vi "CRC.vi"(9 "Len":u8, 11 "u8Buf":u8[](array[numeric]) format="%x") -> (3 "CRC":u16 format="%x")   [LabVIEW 2018]
panel:
  # "CRC-16 Calculation"
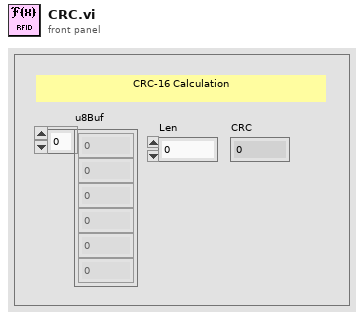
[diagram p1: front panel]
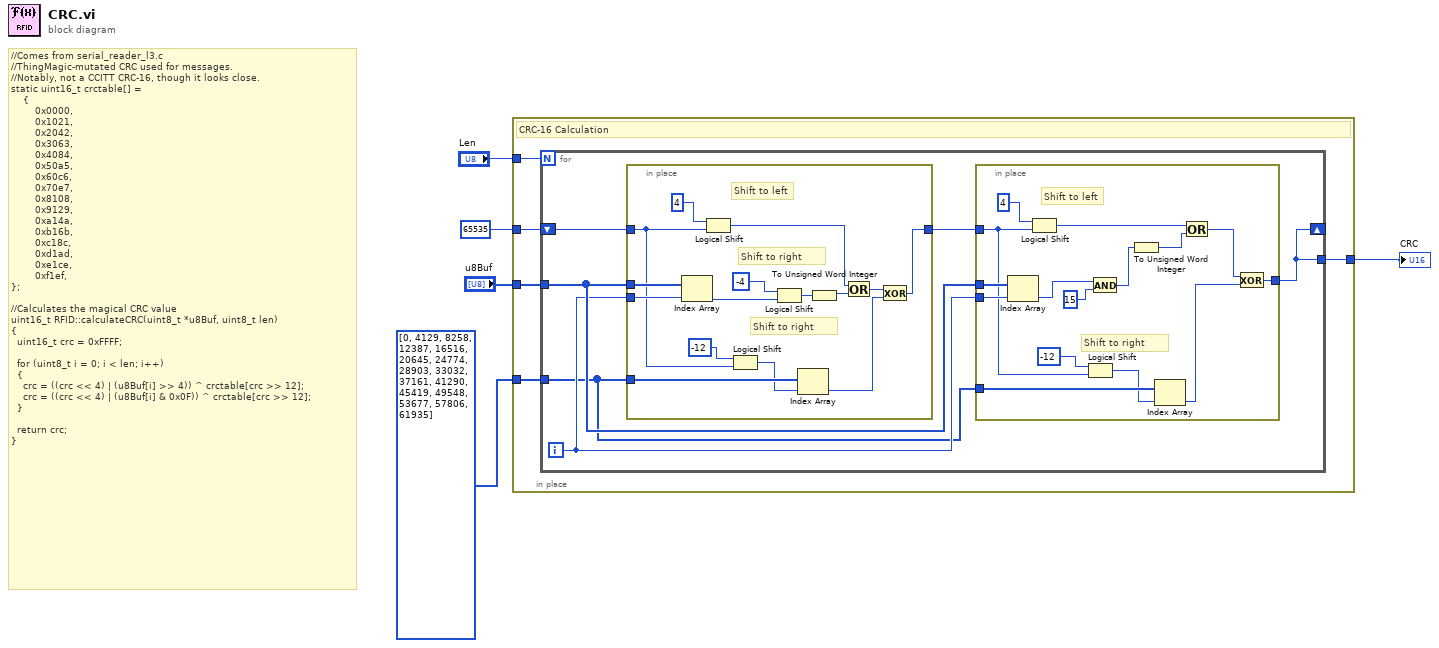
[diagram p0: block diagram]
diagram:
  # "//Comes from serial_reader_l3.c\n//ThingMagic-mutated CRC used for messages.\n//Notably, not a CCITT CRC-16, though it looks close.\nstatic uint16_t crctable[] =\n    {\n        0x0000,\n        0x1021,\n        0x2042,\n        0x3063,\n        0x4084,\n        0x50a5,\n        0x60c6,\n        0x70e7,\n        0x8108,\n        0x9129,\n        0xa14a,\n        0xb16b,\n        0xc18c,\n        0xd1ad,\n        0xe1ce,\n        0xf1ef,\n};\n\n//Calculates the magical CRC value\nuint16_t RFID::calculateCRC(uint8_t *u8Buf, uint8_t len)\n{\n  uint16_t crc = 0xFFFF;\n\n  for (uint8_t i = 0; i < len; i++)\n  {\n    crc = ((crc << 4) | (u8Buf[i] >> 4)) ^ crctable[crc >> 12];\n    crc = ((crc << 4) | (u8Buf[i] & 0x0F)) ^ crctable[crc >> 12];\n  }\n\n  return crc;\n}"
  n1 = in-place {
    in-place-border: "Len" -> [w10]
    in-place-border: u16 65535 -> [w9]
    in-place-border: "u8Buf" -> [w8]
    in-place-border: [w7] -> w2
    in-place-border: u16[] [0, 4129, 8258, 12387, 16516, 20645, 24774, 28903, 33032, 37161, 41290, 45419, 49548, 53677, 57806, 61935] -> [w6]
    # "CRC-16 Calculation"
    n2 = for {
      N: w10 -> [_]
      shift-right: [w11] -> _
      shift-left: w9 -> [w16]
      tunnel: w8 -> [w15]
      tunnel: [w11] -> w7
      tunnel: w6 -> [w13]
      i -> [w14]
      n3 = in-place {
        in-place-border: w15 -> [w45]
        in-place-border: w14 -> [w44]
        in-place-border: w16 -> [w38]
        in-place-border: w13 -> [w40]
        in-place-border: [w32] -> w12
        # "Shift to right"
        # "Shift to right"
        # "Shift to left"
        n4 = Index Array(array=w45, index=w44) -> (element=w42:u8)
        n5 = Logical Shift(y=i16 4, x=w38) -> (x << y=w36:u16)
        n6 = Logical Shift(y=i16 -12, x=w38) -> (x << y=w39:u16)
        n7 = Logical Shift(y=i16 -4, x=w42) -> (x << y=w35:u8)
        n8 = Index Array(array=w40, index=w39) -> (element=w37:u16)
        n9 = To Unsigned Word Integer(number=w35) -> (unsigned 16bit integer=w34:u16)
        n10 = Or(x=w36, y=w34) -> (x .or. y?=w33:u16)
        n11 = Exclusive Or(1:w37, 2:w33) -> (0:w32:u16)
      }
      n12 = in-place {
        in-place-border: w15 -> [w30]
        in-place-border: w14 -> [w29]
        in-place-border: w12 -> [w25]
        in-place-border: w13 -> [w27]
        in-place-border: [w18] -> w11
        # "Shift to right"
        # "Shift to left"
        n13 = Index Array(array=w30, index=w29) -> (element=w24:u8)
        n14 = Logical Shift(y=i16 4, x=w25) -> (x << y=w21:u16)
        n15 = Logical Shift(y=i16 -12, x=w25) -> (x << y=w26:u16)
        n16 = And(x=w24, y=u8 15) -> (x .and. y?=w20:u8)
        n17 = To Unsigned Word Integer(number=w20) -> (unsigned 16bit integer=w19:u16)
        n18 = Index Array(array=w27, index=w26) -> (element=w22:u16)
        n19 = Or(x=w21, y=w19) -> (x .or. y?=w17:u16)
        n20 = Exclusive Or(1:w22, 2:w17) -> (0:w18:u16)
      }
    }
  }
  "CRC" <- w2
